vi "Demo - Test SCPI Message Sequence.vi"() -> ()   [LabVIEW 2020]
panel:
  out "length 6":i32
  out "Response to Start Stream":string
  out "length 5":i32
  out "Response to Voltage DC":string
  out "length 4":i32
  out "Response to Stream Format":string
  out "length 3":i32
  out "Response to Power State":string
  out "length 2":i32
  out "Response to Stop Stream":string
  out "length":i32
  out "Response to System Echo":string
  in  "Port":u16=9760
  in  "IP Address":string="192.168.1.1"
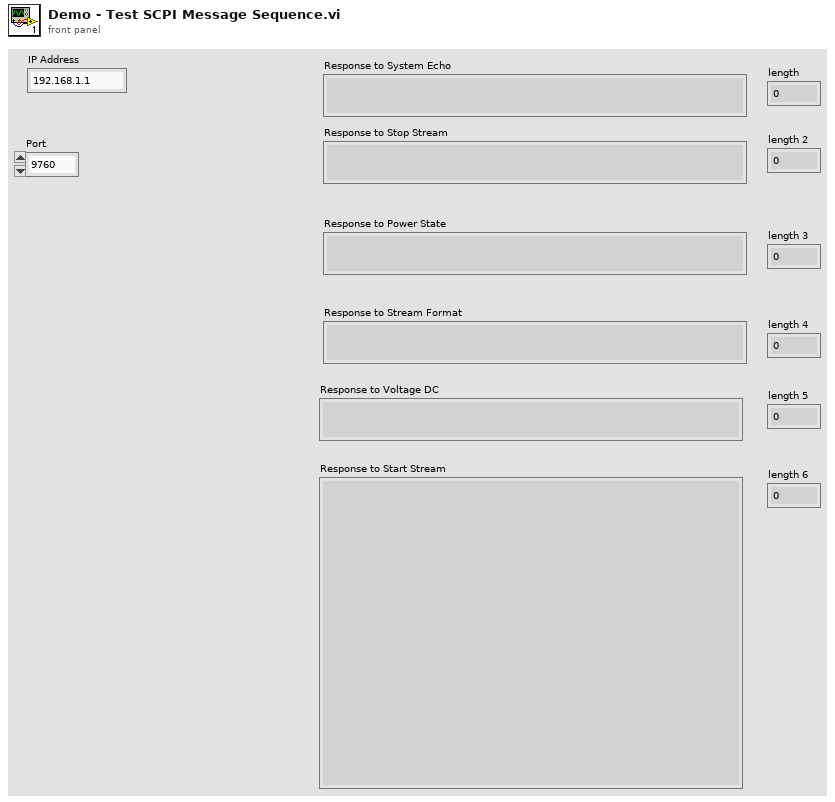
[diagram p1: front panel]
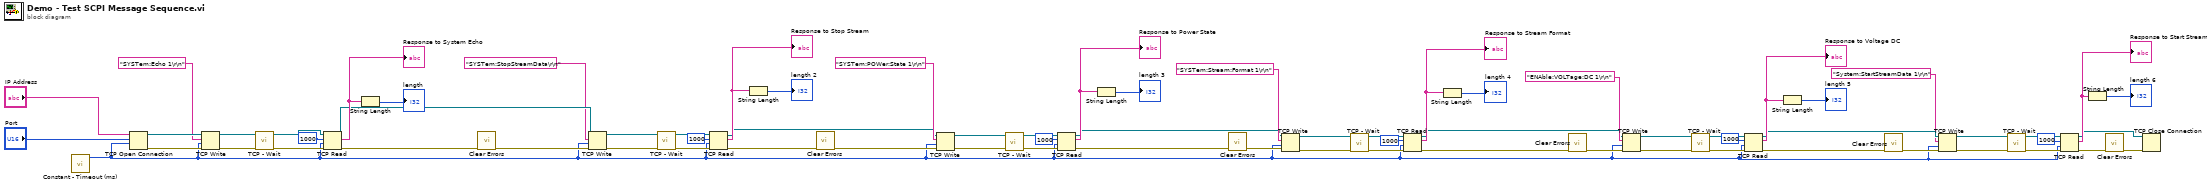
[diagram p0: block diagram]
diagram:
  n1 = call "Constant - Timeout (ms).vi"() -> ("timeout (ms)"=w7:i32)  [unwired: 11 in]
  n2 = TCP Open Connection(address="IP Address", remote port or service name="Port", timeout ms (60000)=w7) -> (connection ID=w69:refnum<k5>, error out=w68:errorcluster)  [unwired: 2 in]
  n3 = TCP Write(connection ID=w69, data in="SYSTem:Echo 1\r\n", error in (no error)=w68, 9:w7) -> (connection ID out=w65:refnum<k5>, error out=w62:errorcluster)  [unwired: 1 out]
  n4 = call "TCP - Wait.vi"("error in"=w62, "TCP Network Connection in"=w65) -> ("error out"=w63:errorcluster, "TCP Network Connection out"=w64:refnum<k5>)  [unwired: 8 in]
  n5 = TCP Read(connection ID=w64, bytes to read=1000, error in (no error)=w63, 9:w7) -> (connection ID out=w59:refnum<k5>, data out=w61:string, error out=w50:errorcluster)  [unwired: 1 in]
  "Response to System Echo" <- w61
  n6 = String Length(string=w61) -> (length=→"length":i32)
  n7 = call <vilib>:"Clear Errors.vi"("error in (no error)"=w50) -> ("error out"=w49:errorcluster)  [unwired: 5 in, 1 out]
  n8 = TCP Write(connection ID=w59, data in="SYSTem:StopStreamData\r\n", error in (no error)=w49, 9:w7) -> (connection ID out=w58:refnum<k5>, error out=w57:errorcluster)  [unwired: 1 out]
  n9 = call "TCP - Wait.vi"("error in"=w57, "TCP Network Connection in"=w58) -> ("error out"=w52:errorcluster, "TCP Network Connection out"=w53:refnum<k5>)  [unwired: 8 in]
  n10 = TCP Read(connection ID=w53, bytes to read=1000, error in (no error)=w52, 9:w7) -> (connection ID out=w38:refnum<k5>, data out=w54:string, error out=w40:errorcluster)  [unwired: 1 in]
  "Response to Stop Stream" <- w54
  n11 = String Length(string=w54) -> (length=→"length 2":i32)
  n12 = call <vilib>:"Clear Errors.vi"("error in (no error)"=w40) -> ("error out"=w39:errorcluster)  [unwired: 5 in, 1 out]
  n13 = TCP Write(connection ID=w38, data in="SYSTem:POWer:State 1\r\n", error in (no error)=w39, 9:w7) -> (connection ID out=w48:refnum<k5>, error out=w47:errorcluster)  [unwired: 1 out]
  n14 = call "TCP - Wait.vi"("error in"=w47, "TCP Network Connection in"=w48) -> ("error out"=w42:errorcluster, "TCP Network Connection out"=w43:refnum<k5>)  [unwired: 8 in]
  n15 = TCP Read(connection ID=w43, bytes to read=1000, error in (no error)=w42, 9:w7) -> (connection ID out=w28:refnum<k5>, data out=w44:string, error out=w27:errorcluster)  [unwired: 1 in]
  "Response to Power State" <- w44
  n16 = String Length(string=w44) -> (length=→"length 3":i32)
  n17 = call <vilib>:"Clear Errors.vi"("error in (no error)"=w27) -> ("error out"=w29:errorcluster)  [unwired: 5 in, 1 out]
  n18 = TCP Write(connection ID=w28, data in="SYSTem:Stream:Format 1\r\n", error in (no error)=w29, 9:w7) -> (connection ID out=w37:refnum<k5>, error out=w36:errorcluster)  [unwired: 1 out]
  n19 = call "TCP - Wait.vi"("error in"=w36, "TCP Network Connection in"=w37) -> ("error out"=w31:errorcluster, "TCP Network Connection out"=w32:refnum<k5>)  [unwired: 8 in]
  n20 = TCP Read(connection ID=w32, bytes to read=1000, error in (no error)=w31, 9:w7) -> (connection ID out=w15:refnum<k5>, data out=w33:string, error out=w16:errorcluster)  [unwired: 1 in]
  "Response to Stream Format" <- w33
  n21 = String Length(string=w33) -> (length=→"length 4":i32)
  n22 = call <vilib>:"Clear Errors.vi"("error in (no error)"=w16) -> ("error out"=w18:errorcluster)  [unwired: 5 in, 1 out]
  n23 = TCP Write(connection ID=w15, data in="ENAble:VOLTage:DC 1\r\n", error in (no error)=w18, 9:w7) -> (connection ID out=w26:refnum<k5>, error out=w25:errorcluster)  [unwired: 1 out]
  n24 = call "TCP - Wait.vi"("error in"=w25, "TCP Network Connection in"=w26) -> ("error out"=w20:errorcluster, "TCP Network Connection out"=w21:refnum<k5>)  [unwired: 8 in]
  n25 = TCP Read(connection ID=w21, bytes to read=1000, error in (no error)=w20, 9:w7) -> (connection ID out=w17:refnum<k5>, data out=w22:string, error out=w14:errorcluster)  [unwired: 1 in]
  "Response to Voltage DC" <- w22
  n26 = String Length(string=w22) -> (length=→"length 5":i32)
  n27 = call <vilib>:"Clear Errors.vi"("error in (no error)"=w14) -> ("error out"=w8:errorcluster)  [unwired: 5 in, 1 out]
  n28 = TCP Write(connection ID=w17, data in="System:StartStreamData 1\r\n", error in (no error)=w8, 9:w7) -> (connection ID out=w13:refnum<k5>, error out=w12:errorcluster)  [unwired: 1 out]
  n29 = call "TCP - Wait.vi"("error in"=w12, "TCP Network Connection in"=w13) -> ("error out"=w10:errorcluster, "TCP Network Connection out"=w11:refnum<k5>)  [unwired: 8 in]
  n30 = TCP Read(connection ID=w11, bytes to read=1000, error in (no error)=w10, 9:w7) -> (connection ID out=w1:refnum<k5>, data out=w4:string, error out=w3:errorcluster)  [unwired: 1 in]
  "Response to Start Stream" <- w4
  n31 = String Length(string=w4) -> (length=→"length 6":i32)
  n32 = call <vilib>:"Clear Errors.vi"("error in (no error)"=w3) -> ("error out"=w2:errorcluster)  [unwired: 5 in, 1 out]
  n33 = TCP Close Connection(connection ID=w1, error in (no error)=w2) -> ()  [unwired: 1 in, 2 out]
